vi "Redo.vi"(7 "Map Model in":refnum<class "Map Model.lvclass">, 8 "error in (no error)":errorcluster, 11 "Set Origin in":refnum<class "Set Origin.lvclass">) -> (0 "error out":errorcluster, 3 "Set Origin out":refnum<class "Set Origin.lvclass">, 5 "Map Model out":refnum<class "Map Model.lvclass">)   [LabVIEW 2020, in "Map Model.lvlib" / "Set Origin.lvclass"]
uses:
  Set Origin.lvclass
  E:/Project/Labview-Projects/Completed projects/Map Editor/Models/Map Model/Tools/Tool/Tool.lvclass
  Map Model/Map Model.lvclass
  Map Model/Map Model.lvclass/Map Model.ctl
  Tool/Tool.lvclass/Tool.ctl
  Tool/Tool.lvclass
panel:
  # "NOTICE -- YOU MUST LEAVE THIS NOTICE IN PLACE.\n\nCopyright (c) 2017, LIANG LIU Shawn.Liu.cn@gmail.com\nAll rights reserved.\n\nRedistribution and use in source and binary forms, with or without modification, are permitted provided that the following conditions are met:\n-Redistributions of source code must retain the above copyright notice, this list of conditions and the following disclaimer.\n-Redistributions in binary form must reproduce the above copyright notice, this list of conditions and the following disclaimer in the documentation and/or other materials provided with the distribution.\n-Neither the name of the eLp nor the names of its contributors may be used to endorse or promote products derived from this software without specific prior written permission.\n\nTHIS SOFTWARE IS PROVIDED BY THE COPYRIGHT HOLDERS AND CONTRIBUTORS \"AS IS\" AND ANY EXPRESS OR IMPLIED WARRANTIES, INCLUDING, BUT NOT LIMITED TO, THE IMPLIED WARRANTIES OF MERCHANTABILITY AND FITNESS FOR A PARTICULAR PURPOSE ARE DISCLAIMED. IN NO EVENT SHALL THE COPYRIGHT HOLDER OR CONTRIBUTORS BE LIABLE FOR ANY DIRECT, INDIRECT, INCIDENTAL, SPECIAL, EXEMPLARY, OR CONSEQUENTIAL DAMAGES (INCLUDING, BUT NOT LIMITED TO, PROCUREMENT OF SUBSTITUTE GOODS OR SERVICES; LOSS OF USE, DATA, OR PROFITS; OR BUSINESS INTERRUPTION) HOWEVER CAUSED AND ON ANY THEORY OF LIABILITY, WHETHER IN CONTRACT, STRICT LIABILITY, OR TORT (INCLUDING NEGLIGENCE OR OTHERWISE) ARISING IN ANY WAY OUT OF THE USE OF THIS SOFTWARE, EVEN IF ADVISED OF THE POSSIBILITY OF SUCH DAMAGE."
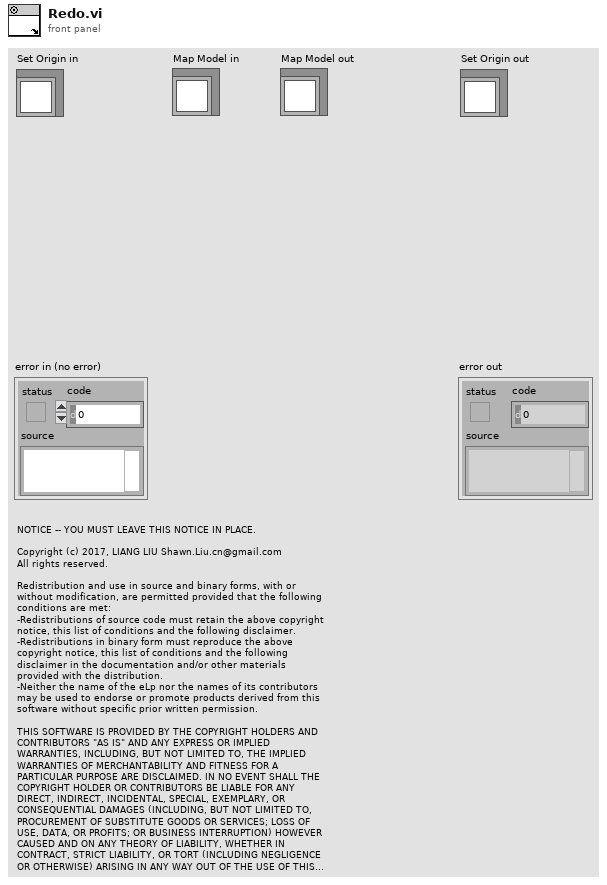
[diagram p1: front panel]
types:
  T1 = typedef "LVPoint32TypeDef.ctl" = cluster{"Horizontal":i32, "Vertical":i32}
  T2 = typedef "LVPointTypeDef.ctl" = cluster{"Horizontal":i16, "Vertical":i16}
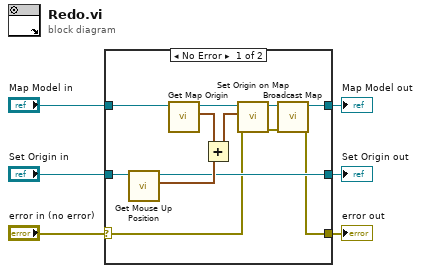
[diagram p0: block diagram]
diagram:
  n1 = case shown="No Error" "error in (no error)" {
    selector: "error in (no error)" -> [w11 w21]
    tunnel: "Map Model in" -> [w15 w20]
    tunnel: "Set Origin in" -> [w13 w19]
    tunnel: [w12 w19] -> w4
    tunnel: [w8 w21] -> w2
    tunnel: [w7 w20] -> w1
    frame No Error {
      n2 = call "Get Mouse Up Position.vi"("Tool in"=w13) -> ("Mouse Up Position"=w14:T1, "Tool out"=w12:refnum<class "Set Origin.lvclass">)  [unwired: 9 in]
      n3 = call "Get Map Origin.vi"("Map Model in"=w15) -> ("Map Origin"=w17:T2, "Map Model out"=w18:refnum<class "Map Model.lvclass">)  [unwired: 9 in]
      n4 = Add(x=w17, y=w14) -> (x+y=w16:T1)
      n5 = call "Set Origin on Map.vi"("error in (no error)"=w11, "Origin on Map"=w16, "Map Model in"=w18) -> ("error out"=w9:errorcluster, "Map Model out"=w10:refnum<class "Map Model.lvclass">)  [unwired: 7 in]
      n6 = call "Broadcast Map.vi"("error in (no error)"=w9, "Map Model in"=w10) -> ("error out"=w8:errorcluster, "Map Model out"=w7:refnum<class "Map Model.lvclass">)  [unwired: 8 in]
    }
    frame Error {
    }
  }
  "error out" <- w2
  "Set Origin out" <- w4
  "Map Model out" <- w1
